vi "ConvertMatlabDataValueToRealNumberOrArrayVariant.vi"(9 "Has Value":bool, 10 "Sizes":i32[](array[numeric]), 11 "Data":dbl[](array[numeric])) -> (3 "Reshaped VArray":variant)   [LabVIEW 2017]
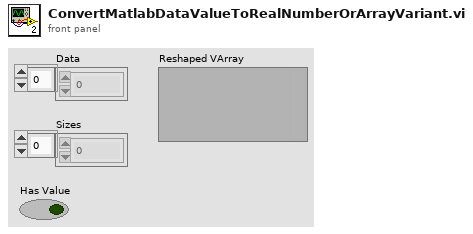
[diagram p1: front panel]
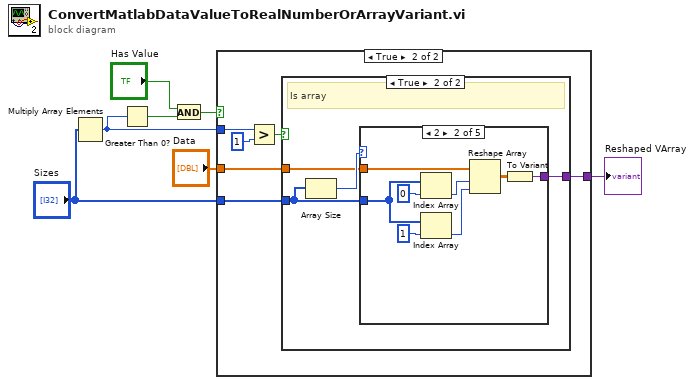
[diagram p0: block diagram]
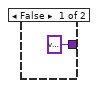
[diagram p2: hidden frame]
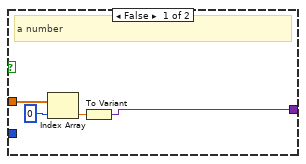
[diagram p3: hidden frame]
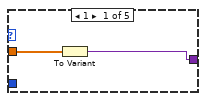
[diagram p4: hidden frame]
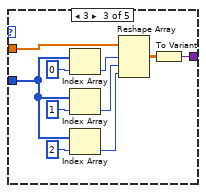
[diagram p5: hidden frame]
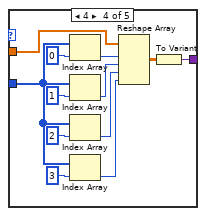
[diagram p6: hidden frame]
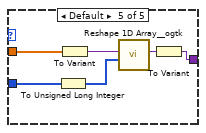
[diagram p7: hidden frame]
diagram:
  n1 = Multiply Array Elements(1:"Sizes") -> (0:w5:i32)
  n2 = Greater Than 0?(x=w5) -> (x > 0?=w4:bool)
  n3 = And(x="Has Value", y=w4) -> (x .and. y?=w7:bool)
  n4 = case shown="True" w7 {
    tunnel: "Sizes" -> [_ w11]
    tunnel: "Data" -> [_ w12]
    tunnel: [variant w10] -> w3
    tunnel: w5 -> [_ w14]
    frame False {
    }
    frame True {
      n5 = Greater?(x=w14, y=1) -> (0:w13:bool)
      n6 = case shown="True" w13 {
        tunnel: w12 -> [w18 w20]
        tunnel: w11 -> [_ w19]
        tunnel: [w15 w21] -> w10
        frame False {
          # "a number"
          n7 = Index Array(array=w18, index=0) -> (element=w16:dbl)
          n8 = To Variant(anything=w16) -> (Variant=w15:variant)
        }
        frame True {
          # "Is array"
          n9 = Array Size(array=w19) -> (size(s)=w22:i32)
          n10 = case shown="2" w22 {
            tunnel: [w23 w25 w33 w43 w59] -> w21
            tunnel: w20 -> [w24 w32 w38 w48 w55]
            tunnel: w19 -> [_ w31 w36 w46 w58]
            frame 1 {
              n11 = To Variant(anything=w24) -> (Variant=w23:variant)
            }
            frame 2 {
              n12 = Index Array(array=w31, index=0) -> (element=w30:i32)
              n13 = Index Array(array=w31, index=1) -> (element=w29:i32)
              n14 = Reshape Array(w32, w30, w29) -> (w26:dbl[][])
              n15 = To Variant(anything=w26) -> (Variant=w25:variant)
            }
            frame 3 {
              n16 = Index Array(array=w36, index=0) -> (element=w42:i32)
              n17 = Index Array(array=w36, index=1) -> (element=w41:i32)
              n18 = Index Array(array=w36, index=2) -> (element=w35:i32)
              n19 = Reshape Array(w38, w42, w41, w35) -> (w34:dbl[][][])
              n20 = To Variant(anything=w34) -> (Variant=w33:variant)
            }
            frame 4 {
              n21 = Index Array(array=w46, index=0) -> (element=w54:i32)
              n22 = Index Array(array=w46, index=1) -> (element=w53:i32)
              n23 = Index Array(array=w46, index=2) -> (element=w49:i32)
              n24 = Index Array(array=w46, index=3) -> (element=w45:i32)
              n25 = Reshape Array(w48, w54, w53, w49, w45) -> (w44:dbl[][][][])
              n26 = To Variant(anything=w44) -> (Variant=w43:variant)
            }
            frame Default {
              n27 = To Unsigned Long Integer(number=w58) -> (unsigned 32bit integer=w57:u32[])
              n28 = To Variant(anything=w55) -> (Variant=w56:variant)
              n29 = call <userlib>:"Reshape 1D Array__ogtk.vi"("Size(s)"=w57, "1D Array"=w56) -> ("Reshaped VArray"=w60:variant)  [unwired: 8 in, 1 out]
              n30 = To Variant(anything=w60) -> (Variant=w59:variant)
            }
          }
        }
      }
    }
  }
  "Reshaped VArray" <- w3
